vi "test4.3-AsyncMessageWithoutReply_Queue.vi"(8 "error in (no error)":errorcluster, 11 "TestCase in":refnum<class "testcase-CSMGlobalLog.lvclass">) -> (0 "error out":errorcluster, 3 "TestCase out":refnum<class "testcase-CSMGlobalLog.lvclass">)   [LabVIEW 2017, in "testcase-CSMGlobalLog.lvclass"]
uses:
  testcase-CSMGlobalLog.lvclass
  testcase-CSMGlobalLog.lvclass/testcase-CSMGlobalLog.ctl
  c9cb4a92-c6b2-48ff-9945-b938079fd949.vi
  <vilib>/addons/_JKI Toolkits/VI Tester/TestCase.llb/TestCase.lvclass
  src/user.lib/_NEVSTOP/Communicable State Machine(CSM)/Communicable State Machine.lvlib
  src/user.lib/_NEVSTOP/Communicable State Machine(CSM)/Utility/Periodic String Filter Setting.ctl
  CSM/CSM-Testcase.lvlib
  C:/Program Files (x86)/National Instruments/LabVIEW 2017/vi.lib/addons/_JKI Toolkits/VI Tester/TestCase.llb/TestCase.lvclass
panel:
  out "String cache total":string
  out "LoopCount":i32
  out "String Cache each loop":string
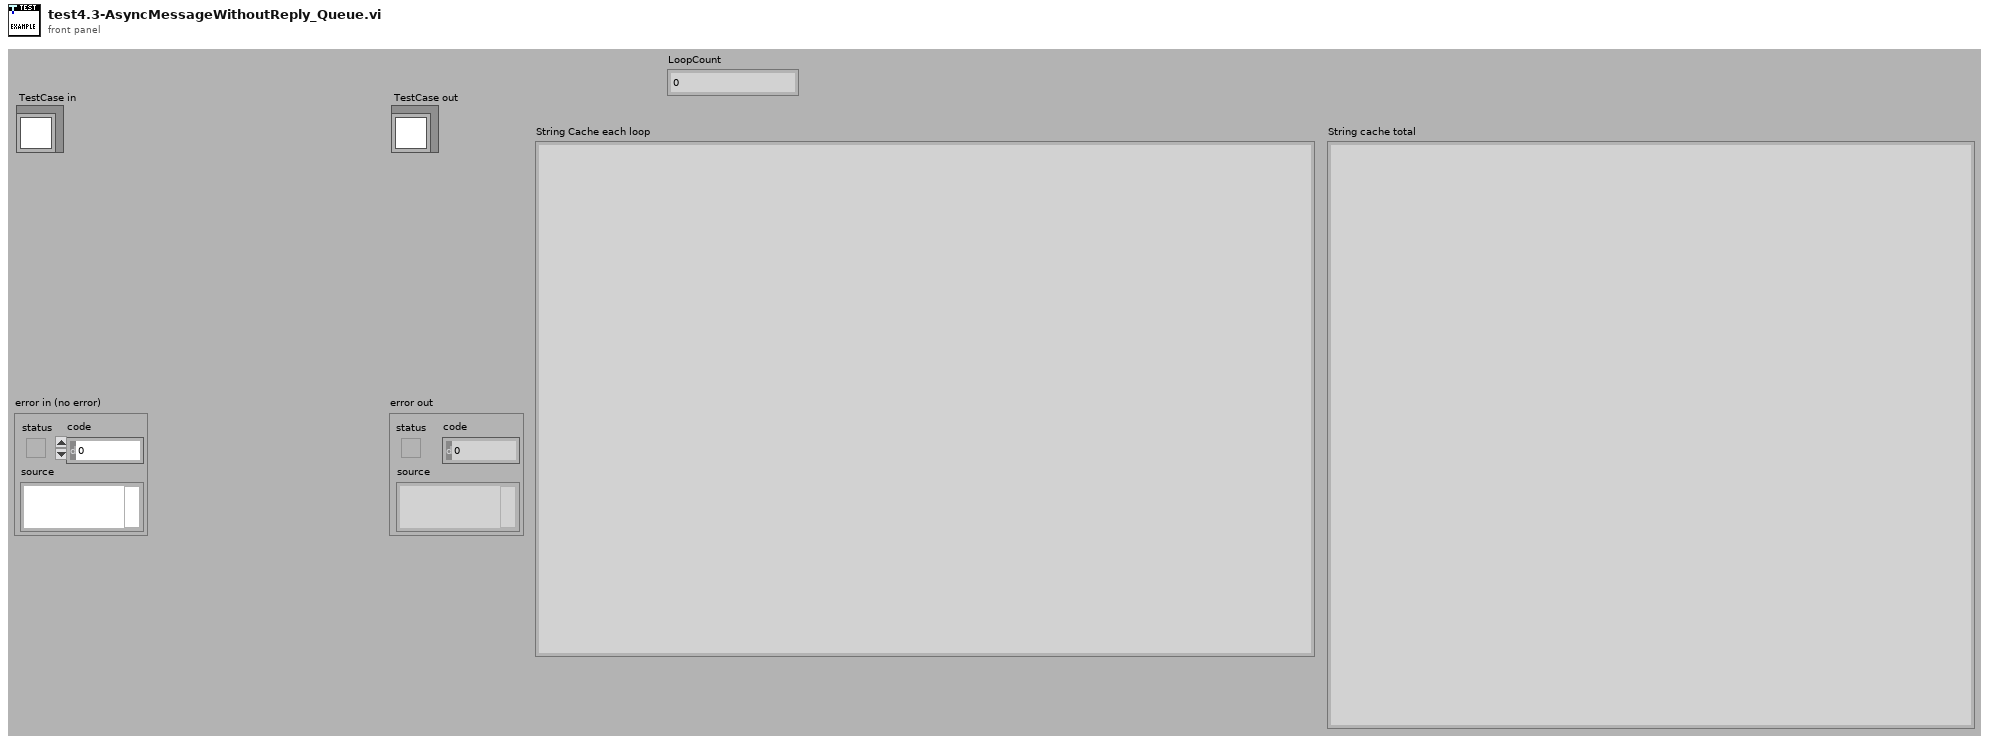
[diagram p1: front panel]
types:
  T1 = typedef "Communicable State Machine.lvlib/Periodic String Filter Setting.ctl" = cluster{"threashold(#/s)":dbl, "Check Peroid(s)":dbl}
  T2 = typedef "Communicable State Machine.lvlib/_CSM_GlobalLog_MSG.ctl" = cluster{"Name (\"\" to Use UUID)":string, "Current State":string, "Arguments":string, "Source Message":T3, "Source Module":string, "Complete(T)/Start(F)":bool, "LogType":T4, "Time Stamp":timestamp}
  T3 = typedef "Communicable State Machine.lvlib/_CSM_Response Source Message.ctl" = cluster{"‘State":string, "’Arguments":string, "’Error":errorcluster}
  T4 = typedef "Communicable State Machine.lvlib/_CSM_GlobalLog_MSG_TYPE.ctl" = enum16{"User Log", "State Change", "Status", "Interrupt", "Register", "Unregister", "Error Log", "Module Created", "Module Destroyed", "Async Message", "No-Rep Async Message", "Sync Message"}
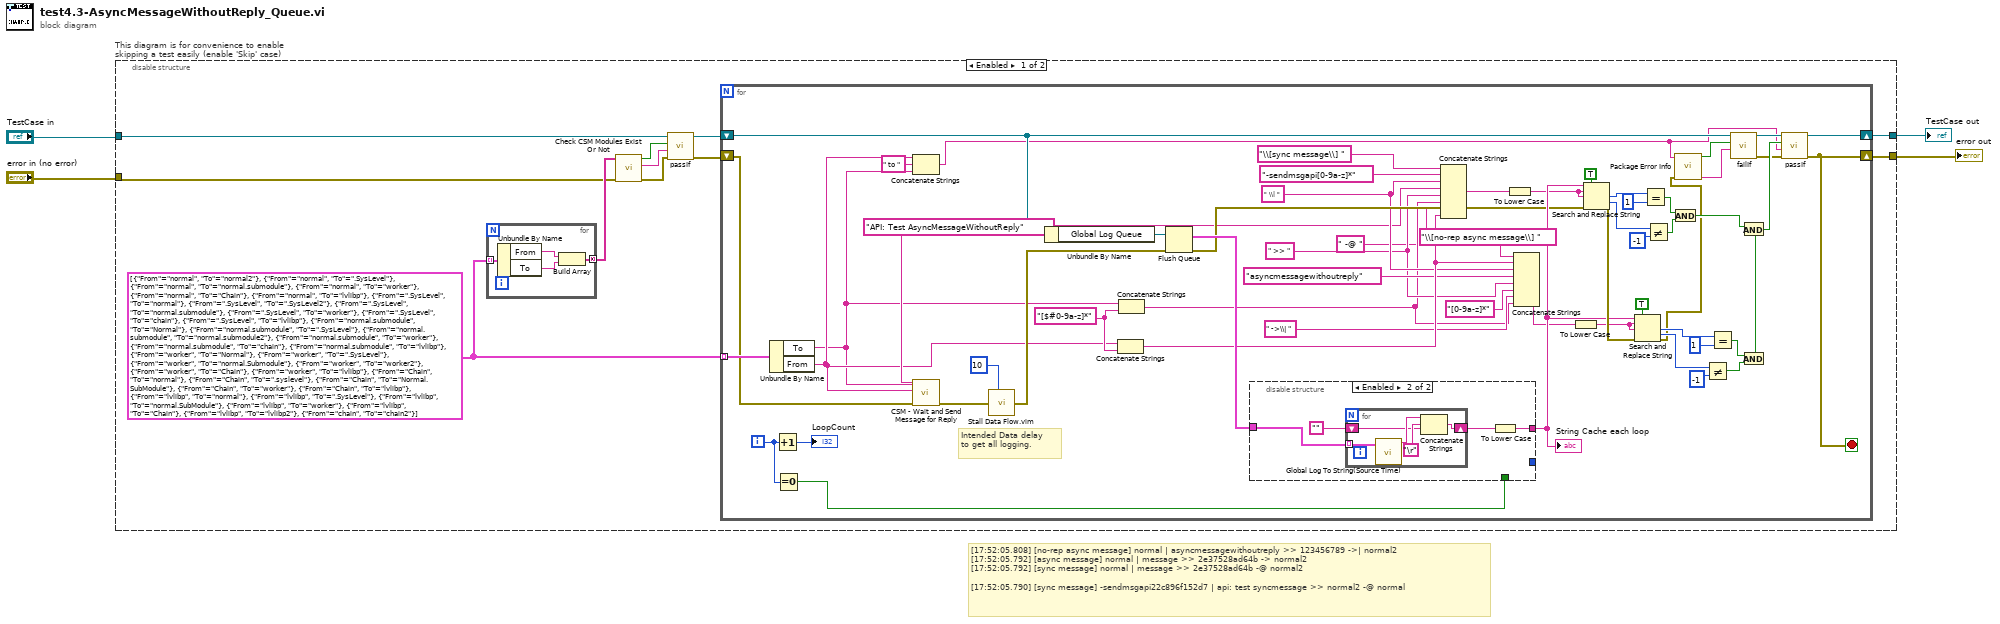
[diagram p0: block diagram]
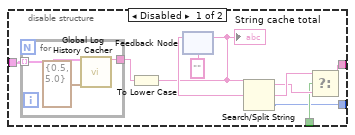
[diagram p2: hidden frame]
diagram:
  # "[17:52:05.808] [no-rep async message] normal | asyncmessagewithoutreply >> 123456789 ->| normal2\n[17:52:05.792] [async message] normal | message >> 2e37528ad64b -> normal2\n[17:52:05.792] [sync message] normal | message >> 2e37528ad64b -@ normal2\n\n[17:52:05.790] [sync message] -sendmsgapi22c896f152d7 | api: test syncmessage >> normal2 -@ normal"
  n1 = disable-structure "This diagram is for convenience to enable skipping a test easily (enable 'Skip' case)" shown="Enabled" {
    disable-tunnel: "TestCase in" -> [w8 w104]
    disable-tunnel: [w14 w102] -> w1
    disable-tunnel: [w15 w103] -> w3
    disable-tunnel: "error in (no error)" -> [w5 w101]
    frame Enabled {
      w9 = cluster{"From":string, "To":string}[] [{"From"="normal", "To"="normal2"}, {"From"="normal", "To"=".SysLevel"}, {"From"="normal", "To"="normal.submodule"}, {"From"="normal", "To"="worker"}, {"From"="normal", "To"="Chain"}, {"From"="normal", "To"="lvlibp"}, {"From"=".SysLevel", "To"="normal"}, {"From"=".SysLevel", "To"=".SysLevel2"}, {"From"=".SysLevel", "To"="normal.submodule"}, {"From"=".SysLevel", "To"="worker"}, {"From"=".SysLevel", "To"="chain"}, {"From"=".SysLevel", "To"="lvlibp"}, {"From"="normal.submodule", "To"="Normal"}, {"From"="normal.submodule", "To"=".SysLevel"}, {"From"="normal.submodule", "To"="normal.submodule2"}, {"From"="normal.submodule", "To"="worker"}, {"From"="normal.submodule", "To"="chain"}, {"From"="normal.submodule", "To"="lvlibp"}, {"From"="worker", "To"="Normal"}, {"From"="worker", "To"=".SysLevel"}, {"From"="worker", "To"="normal.Submodule"}, {"From"="worker", "To"="worker2"}, {"From"="worker", "To"="Chain"}, {"From"="worker", "To"="lvlibp"}, {"From"="Chain", "To"="normal"}, {"From"="Chain", "To"=".syslevel"}, {"From"="Chain", "To"="Normal.SubModule"}, {"From"="Chain", "To"="worker"}, {"From"="Chain", "To"="lvlibp"}, {"From"="lvlibp", "To"="normal"}, {"From"="lvlibp", "To"=".SysLevel"}, {"From"="lvlibp", "To"="normal.SubModule"}, {"From"="lvlibp", "To"="worker"}, {"From"="lvlibp", "To"="Chain"}, {"From"="lvlibp", "To"="lvlibp2"}, {"From"="chain", "To"="chain2"}]
      n2 = for {
        tunnel: w9 -> [w19] mode=indexing
        tunnel: [w16] -> w12 mode=concatenating
        n3 = Unbundle By Name(w19) -> ("From"=w18:string, "To"=w17:string)
        n4 = Build Array(w18, w17) -> (w16:string[])
      }
      n5 = call "Check CSM Modules Exist Or Not.vi"("error in"=w5, "CSM names in"=w12) -> ("error out"=w10:errorcluster, "Debug string"=w11:string, "All Modules Exist?"=w13:bool)  [unwired: 7 in]
      n6 = call-dynamic "passIf.vi"("error in (no error)"=w10, "message (\"\")"=w11, "pass"=w13, "TestCase in"=w8) -> ("error out"=w6:errorcluster, "TestCase out"=w7:refnum<class "testcase-CSMGlobalLog.lvclass">)  [unwired: 6 in]
      n7 = for {
        tunnel: w9 -> [w58] mode=indexing
        shift-right: [w57] -> w15
        shift-left: w6 -> [w30]
        shift-right: [w78] -> w14
        shift-left: w7 -> [w27]
        i -> [w56]
        stop <- w57 stop-if-true
        w32 = "[$#0-9a-z]*" ("string")
        w42 = " >> "
        w44 = " \\| "
        w34 = "API: Test AsyncMessageWithoutReply" ("State")
        # "Intended Data delay\nto get all logging."
        n8 = Unbundle By Name(w58) -> ("To"=w22:string, "From"=w23:string)
        n9 = Increment(x=w56) -> (x+1=→"LoopCount":i32)
        n10 = Equal To 0?(x=w56) -> (x = 0?=w49:bool)
        n11 = Concatenate Strings(w23, " to " ("string"), w22) -> (w20:string)
        n12 = call "CSM - Wait and Send Message for Reply.vi"("State"=w34, "Arguments (\"\")"=w22, "Target Module"=w23, "Error In (No Error)"=w30) -> ("error out"=w55:errorcluster)  [unwired: 8 in, 3 out]
        n13 = call "Stall Data Flow.vim"("value in"=w55, "milliseconds to wait"=u32 10 ("millisecond timer value")) -> ("value out"=w54:errorcluster)  [unwired: 1 out]
        n14 = Unbundle By Name(w27) -> ("Global Log Queue"=w77:refnum<queue>)
        n15 = Concatenate Strings(w23, w32) -> (w45:string)
        n16 = Concatenate Strings(w22, w32) -> (w39:string)
        n17 = Flush Queue(queue=w77, error in (no error)=w54) -> (remaining elements=w51:T2[], error out=w48:errorcluster)  [unwired: 1 out]
        n18 = disable-structure shown="Enabled" {
          disable-tunnel: [w82 w92] -> w50
          disable-tunnel: w49 -> [w81 _]
          disable-tunnel: w51 -> [w80 w94]
          disable-tunnel: [w79 _] -> _
          frame Disabled {
            n19 = for {
              tunnel: w80 -> [w91] mode=indexing
              tunnel: [w90] -> w88
              n20 = call "Global Log History Cacher.vi"("Global Log Data"=w91, "Settings"=T1 {"threashold(#/s)"=0.5, "Check Peroid(s)"=5.0}) -> ("String Cache"=w90:string)  [unwired: 13 in]
            }
            n21 = To Lower Case(string=w88) -> (all lower case string=w83:string)
            "String cache total" <- w83
            n22 = feedback #1("") -> (w87:string)
            n23 = feedback-in #1(w83) -> ()
            n24 = Search/Split String(string=w83, search string/char (-)=w87) -> (substring before match=w84:string, match + rest of string=w85:string, offset of match=w79:i32)  [unwired: 1 in]
            n25 = Select(t=w85, s=w81, f=w84) -> (s? t:f=w82:string)
          }
          frame Enabled {
            n26 = for {
              tunnel: w94 -> [w100] mode=indexing
              shift-right: [w96] -> w93
              shift-left: "" -> [w97]
              n27 = call "Global Log To String(Source Time).vi"("Log"=w100) -> ("Log String"=w99:string)  [unwired: 9 in]
              n28 = Concatenate Strings(w99, "\r", w97) -> (w96:string)
            }
            n29 = To Lower Case(string=w93) -> (all lower case string=w92:string)
          }
        }
        "String Cache each loop" <- w50
        n30 = Concatenate Strings("\\[sync message\\] ", "-sendmsgapi[0-9a-z]*", w44, w34, w42, w39, " -@ " ("string"), w45) -> (w38:string)
        n31 = To Lower Case(string=w38) -> (all lower case string=w37:string)
        n32 = Concatenate Strings("\\[no-rep async message\\] " ("string"), w45, w44, "asyncmessagewithoutreply", w42, "[0-9a-z]*", " ->\\| ", w39) -> (w36:string)
        n33 = To Lower Case(string=w36) -> (all lower case string=w35:string)
        n34 = Search and Replace String(replace all?=TRUE ("replace all? (F)"), input string=w50, search string=w37, replace string=w37, error in=w48) -> (number of replacements=w74:i32, offset past replacement=w73:i32, error out=w63:errorcluster)  [unwired: 3 in, 1 out]
        n35 = Search and Replace String(replace all?=TRUE ("replace all? (F)"), input string=w50, search string=w35, replace string=w35, error in=w63) -> (number of replacements=w65:i32, offset past replacement=w66:i32, error out=w24:errorcluster)  [unwired: 3 in, 1 out]
        n36 = Equal?(x=w74, y=1) -> (x = y?=w71:bool)
        n37 = Not Equal?(x=w73, y=-1) -> (x != y?=w70:bool)
        n38 = And(x=w71, y=w70) -> (x .and. y?=w59:bool)
        n39 = call "Package Error Info.vi"("error in"=w24, "String in"=w20) -> ("packed error info out"=w28:string, "error status"=w29:bool)  [unwired: 8 in]
        n40 = Not Equal?(x=w66, y=-1) -> (x != y?=w69:bool)
        n41 = Equal?(x=w65, y=1) -> (x = y?=w68:bool)
        n42 = call-dynamic "failIf.vi"("message (\"\")"=w28, "fail"=w29, "TestCase in"=w27) -> ("error out"=w25:errorcluster, "TestCase out"=w26:refnum<class "testcase-CSMGlobalLog.lvclass">)  [unwired: 7 in]
        n43 = And(x=w68, y=w69) -> (x .and. y?=w62:bool)
        n44 = And(x=w59, y=w62) -> (x .and. y?=w52:bool)
        n45 = call-dynamic "passIf.vi"("error in (no error)"=w25, "message (\"\")"=w20, "pass"=w52, "TestCase in"=w26) -> ("error out"=w57:errorcluster, "TestCase out"=w78:refnum<class "testcase-CSMGlobalLog.lvclass">)  [unwired: 6 in]
      }
    }
    frame Disabled {
      # "skip test result while test is under development"
      n46 = call <vilib>:"skip.vi"("error in (no error)"=w101, "TestCase in"=w104) -> ("error out"=w103:errorcluster, "TestCase out"=w102:refnum<class "testcase-CSMGlobalLog.lvclass">)  [unwired: 8 in]
    }
  }
  "error out" <- w3
  "TestCase out" <- w1
